vi "数据库读取B.vi"() -> (1 "当日合格数":i32, 2 "当天总数":i32, 3 "Data":string[][](array[string]))   [LabVIEW 2014]
panel:
  out "error out 2":errorcluster
  out "error out":errorcluster
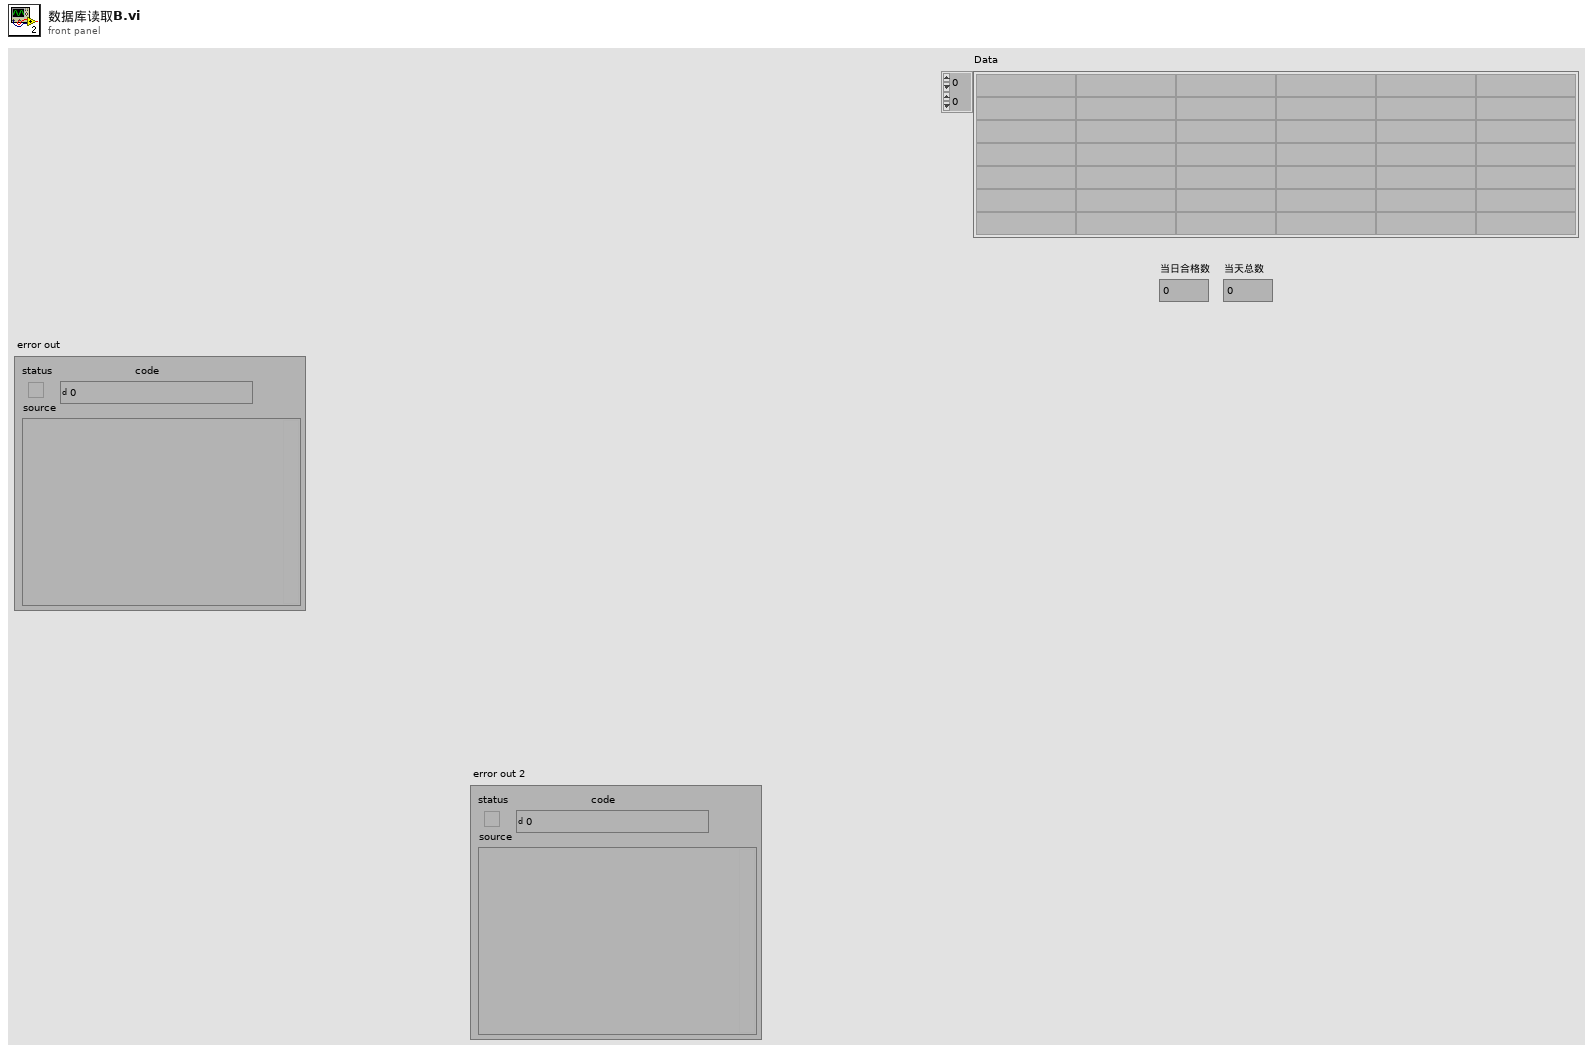
[diagram p1: front panel]
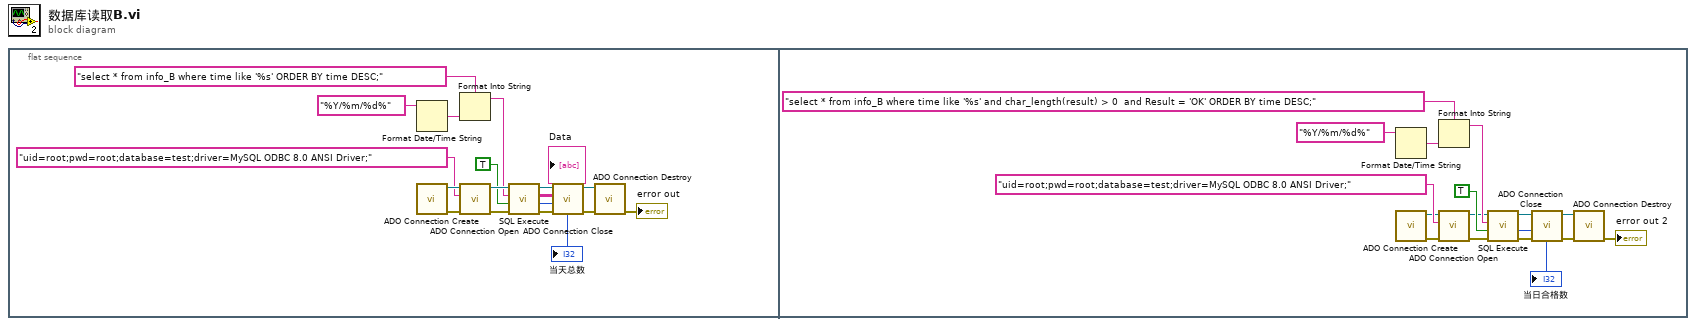
[diagram p0: block diagram]
diagram:
  n1 = flat-sequence {
    frame #0 {
      n2 = Format Date/Time String(time format string (%c)="%Y/%m/%d%" ("时间格式字符串(%c)")) -> (date/time string=w5:string)  [unwired: 2 in]
      n3 = call "ADO Connection Create.vi"() -> ("error out"=w16:errorcluster, "ADODB._Connection Out"=w17:refnum<k7>)  [unwired: 10 in]
      n4 = Format Into String(format string="select * from info_B where time like '%s' ORDER BY time DESC;" ("Command Text"), w5) -> (resulting string=w3:string)  [unwired: 2 in, 1 out]
      n5 = call "ADO Connection Open.vi"("error in (no error)"=w16, "ConnectionString"="uid=root;pwd=root;database=test;driver=MySQL ODBC 8.0 ANSI Driver;", "ADODB._Connection In"=w17) -> ("error out"=w14:errorcluster, "ADODB._Connection Out"=w15:refnum<k7>)  [unwired: 7 in]
      n6 = call "SQL Execute.vi"("error in (no error)"=w14, "Return Data (T)"=TRUE, "Command Text"=w3, "ADODB._Connection In"=w15) -> ("error out"=w12:errorcluster, "Rows Fetched"=→"当天总数":i32, "Data"=→"Data":string[][], "ADODB._Connection Out"=w13:refnum<k7>)  [unwired: 4 in]
      n7 = call "ADO Connection Close.vi"("error in (no error)"=w12, "ADODB._Connection In"=w13) -> ("error out"=w10:errorcluster, "ADODB._Connection Out"=w11:refnum<k7>)  [unwired: 8 in]
      n8 = call "ADO Connection Destroy.vi"("error in (no error)"=w10, "ADODB._Connection In"=w11) -> ("error out"=→"error out":errorcluster)  [unwired: 9 in]
    }
    frame #1 {
      n9 = Format Date/Time String(time format string (%c)="%Y/%m/%d%" ("时间格式字符串(%c)")) -> (date/time string=w31:string)  [unwired: 2 in]
      n10 = call "ADO Connection Create.vi"() -> ("error out"=w20:errorcluster, "ADODB._Connection Out"=w19:refnum<k7>)  [unwired: 10 in]
      n11 = Format Into String(format string="select * from info_B where time like '%s' and char_length(result) > 0  and Result = 'OK' ORDER BY time DESC;" ("Command Text"), w31) -> (resulting string=w33:string)  [unwired: 2 in, 1 out]
      n12 = call "ADO Connection Open.vi"("error in (no error)"=w20, "ConnectionString"="uid=root;pwd=root;database=test;driver=MySQL ODBC 8.0 ANSI Driver;", "ADODB._Connection In"=w19) -> ("error out"=w22:errorcluster, "ADODB._Connection Out"=w21:refnum<k7>)  [unwired: 7 in]
      n13 = call "SQL Execute.vi"("error in (no error)"=w22, "Return Data (T)"=TRUE, "Command Text"=w33, "ADODB._Connection In"=w21) -> ("error out"=w24:errorcluster, "Rows Fetched"=→"当日合格数":i32, "ADODB._Connection Out"=w23:refnum<k7>)  [unwired: 4 in, 1 out]
      n14 = call "ADO Connection Close.vi"("error in (no error)"=w24, "ADODB._Connection In"=w23) -> ("error out"=w26:errorcluster, "ADODB._Connection Out"=w25:refnum<k7>)  [unwired: 8 in]
      n15 = call "ADO Connection Destroy.vi"("error in (no error)"=w26, "ADODB._Connection In"=w25) -> ("error out"=→"error out 2":errorcluster)  [unwired: 9 in]
    }
  }
